vi "Create File Named by DataTime.vi"(8 "error in (no error)":errorcluster, 10 "suffix":string, 11 "prefix":string) -> (0 "error out":errorcluster, 3 "Byte Stream File out":refnum<file>)   [LabVIEW 2016, in "Common.lvlib"]
uses:
  <userlib>/Common Components/Common/Common.lvlib
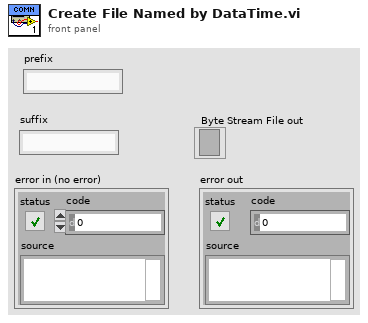
[diagram p1: front panel]
types:
  T1 = enum16{"open", "replace", "create", "open or create", "replace or create", "replace or create with confirmation"}
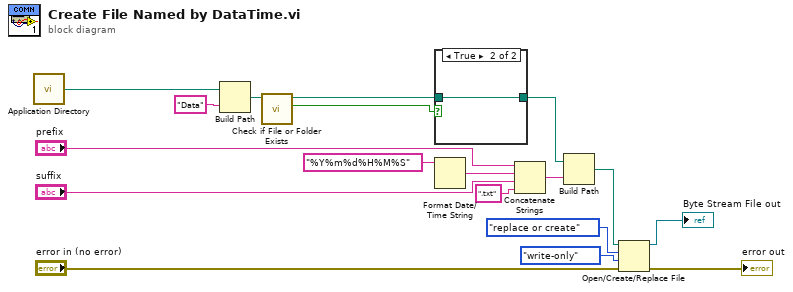
[diagram p0: block diagram]
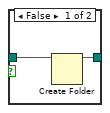
[diagram p2: hidden frame]
diagram:
  n1 = call <vilib>:"Application Directory.vi"() -> ("Application Directory"=w11:path)
  n2 = Build Path(base path=w11, name or relative path="Data") -> (appended path=w10:path)
  n3 = call <vilib>:"Check if File or Folder Exists.vi"("path"=w10) -> ("file or folder exists?"=w8:bool, "dup path"=w7:path)  [unwired: 8 in, 1 out]
  n4 = case shown="True" w8 {
    tunnel: w7 -> [w20 w21]
    tunnel: [w19 w21] -> w6
    frame False {
      n5 = Create Folder(path (use dialog)=w20) -> (created path=w19:path)  [unwired: 2 in, 2 out]
    }
    frame True {
    }
  }
  n6 = Format Date/Time String(time format string (%c)="%Y%m%d%H%M%S") -> (date/time string=w5:string)  [unwired: 2 in]
  n7 = Concatenate Strings("prefix", w5, "suffix", ".txt") -> (w2:string)
  n8 = Build Path(base path=w6, name or relative path=w2) -> (appended path=w13:path)
  n9 = Open/Create/Replace File(file path (use dialog)=w13, error in="error in (no error)", operation (0:open)=T1."replace or create", access (0:read/write)=enum16{"read/write", "read-only", "write-only"}."write-only") -> (refnum out=→"Byte Stream File out":refnum<file>, error out=→"error out":errorcluster)  [unwired: 2 in, 1 out]
